vi "współrzedne geograficzne na UTM.vi"(0 "Położenie robota - długość geograficzna":dbl=44.0 format="%#_19g", 2 "Położenie robota - szerokość geograficzna":dbl=73.0 format="%#_19g", 3 "a":dbl=6378137.0 format="%_20g", 5 "b":dbl=6356752.3142452 format="%_20f") -> (6 "Strefa":string, 7 "E":dbl format="%.20g", 8 "N":dbl format="%.20g")   [LabVIEW 2015, in "Biblioteka moduł map v3.lvlib" / "Konwersja wsp.lvlib" / "UTM.lvlib"]
doc: "Jako argumenty przyjmowane są współrzędne w stopniach dziesiętnych. Domyslnie konwersja jest dokonywana dla współrzędnych w odwzorowaniu WGS84. Chcąc zastosować inne odwzorowanie Ziemi należy zmienić parametry geoidy (a,b).\nNa wyjscciu otrzymujemy strefę w pozycjonowaniu UTM oraz położenie N i E ( nie są to odpowiedniki kierunku północ, wschód). \n\nNie uwzględnoine zostały nierównomierne strefy: 31X, 33X, 35X, 37X, 31V, 32V dlatego dla tych obszarów nie powinno się stosować tego algorytmu. Dodatkowo nie wolno go stosować dla współrzędnych geograficznych znajdujących się poza zakresem 84 stopni N i 80 stopni S."
uses:
  UTM.lvlib
  Konwersja na UTM/Konwersja na UTM.lvlib
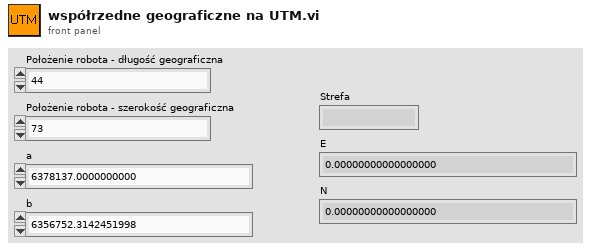
[diagram p1: front panel]
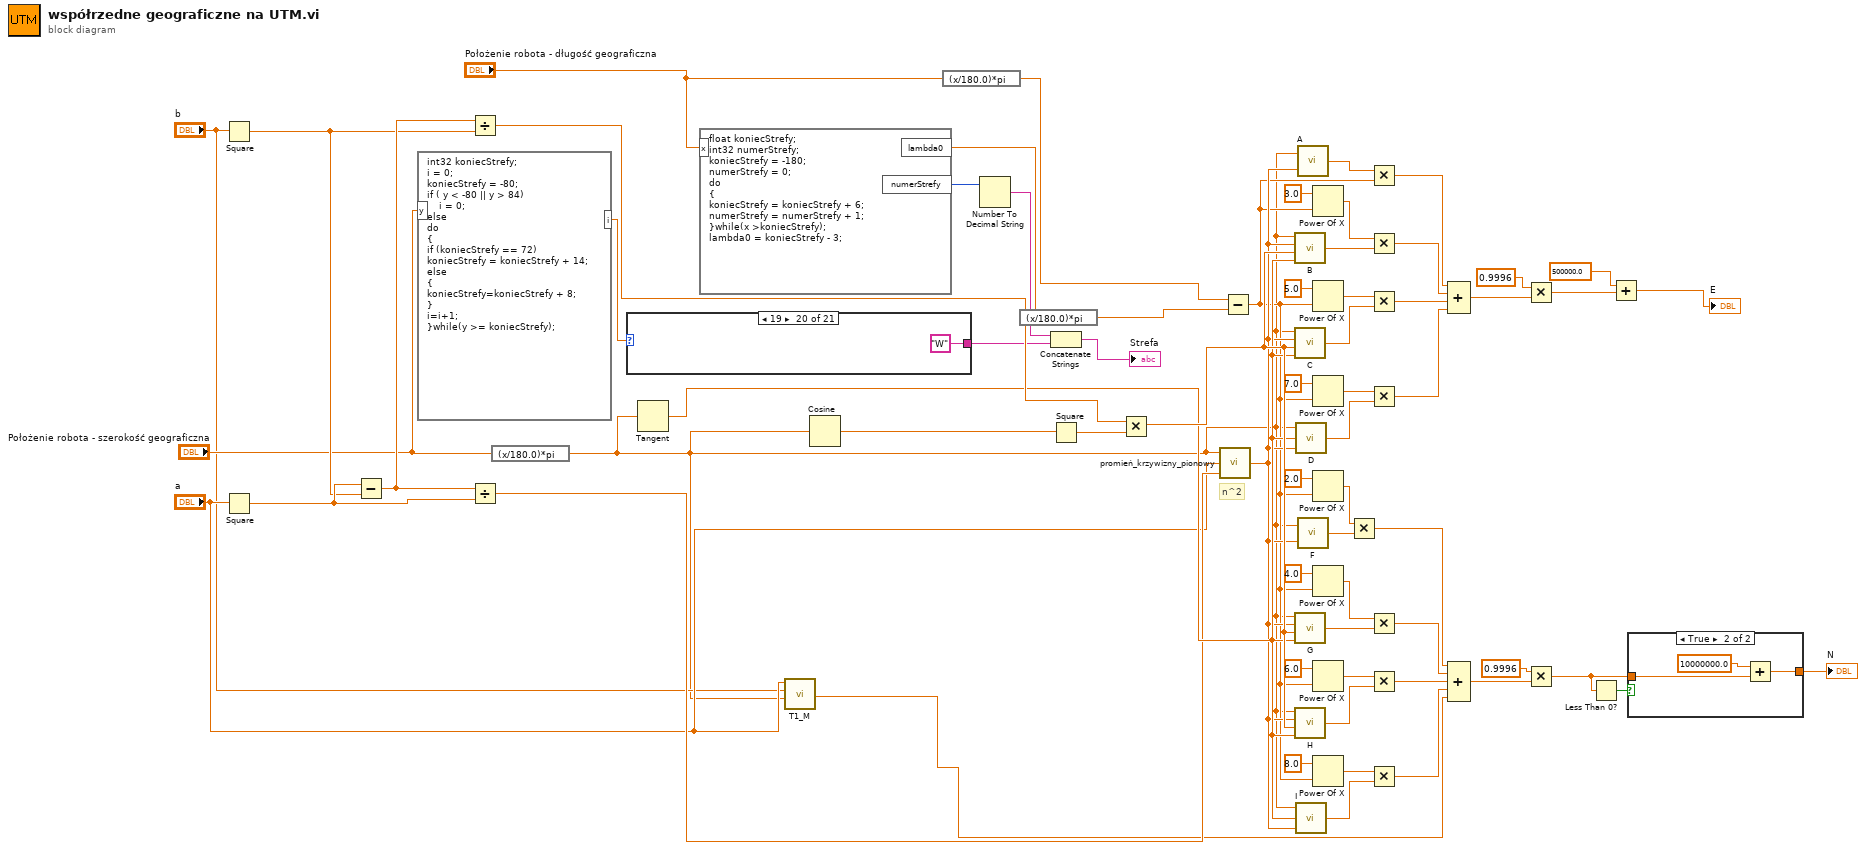
[diagram p0: block diagram]
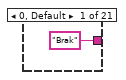
[diagram p3: hidden frame]
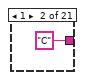
[diagram p4: hidden frame]
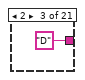
[diagram p5: hidden frame]
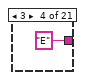
[diagram p6: hidden frame]
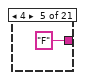
[diagram p7: hidden frame]
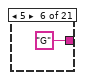
[diagram p8: hidden frame]
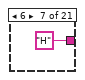
[diagram p9: hidden frame]
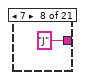
[diagram p10: hidden frame]
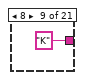
[diagram p11: hidden frame]
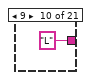
[diagram p12: hidden frame]
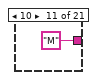
[diagram p13: hidden frame]
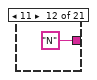
[diagram p14: hidden frame]
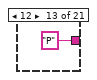
[diagram p15: hidden frame]
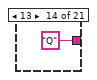
[diagram p16: hidden frame]
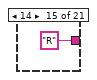
[diagram p17: hidden frame]
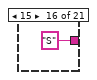
[diagram p18: hidden frame]
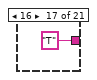
[diagram p19: hidden frame]
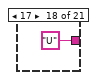
[diagram p20: hidden frame]
diagram:
  # "n^2"
  n1 = Square(x="b") -> (x^2=w63:dbl)
  n2 = Square(x="a") -> (x^2=w64:dbl)
  n3 = Subtract(x=w64, y=w63) -> (x-y=w65:dbl)
  n4 = formula code="int32 koniecStrefy;\ni = 0;\nkoniecStrefy = -80;\nif ( y < -80 || y > 84)\n    i = 0;\nelse\ndo\n{\nif (koniecStrefy == 72)\nkoniecStrefy = koniecStrefy + 14;\nelse\n{\nkoniecStrefy=koniecStrefy + 8;\n}\ni=i+1;\n}while(y >= koniecStrefy);"("y"="Położenie robota - szerokość geograficzna") -> ("i"=w16:dbl)
  n5 = Divide(x=w65, y=w63) -> (x/y=w60:dbl)
  n6 = Divide(x=w65, y=w64) -> (x/y=w54:dbl)
  n7 = expression code="(x/180.0)*pi" ("degrees to radians")("Położenie robota - szerokość geograficzna") -> (w2:dbl)
  n8 = case shown="19" w16 {
    tunnel: ["Brak" "C" "D" "E" "F" "G" "H" "J" "K" "L" "M" "N" "P" "Q" "R" "S" "T" "U" "V" "W" "X"] -> w14
    frame 0, Default {
    }
    frame 1 {
    }
    frame 2 {
    }
    frame 3 {
    }
    frame 4 {
    }
    frame 5 {
    }
    frame 6 {
    }
    frame 7 {
    }
    frame 8 {
    }
    frame 9 {
    }
    frame 10 {
    }
    frame 11 {
    }
    frame 12 {
    }
    frame 13 {
    }
    frame 14 {
    }
    frame 15 {
    }
    frame 16 {
    }
    frame 17 {
    }
    frame 18 {
    }
    frame 19 {
    }
    frame 20 {
    }
  }
  n9 = Tangent(1:w2) -> (0:w56:dbl)
  n10 = formula code="float koniecStrefy;\nint32 numerStrefy;\nkoniecStrefy = -180;\nnumerStrefy = 0;\ndo\n{\nkoniecStrefy = koniecStrefy + 6;\nnumerStrefy = numerStrefy + 1;\n}while(x >koniecStrefy);\nlambda0 = koniecStrefy - 3;"("x"="Położenie robota - długość geograficzna") -> ("lambda0"=w24:dbl, "numerStrefy"=w15:i32)
  n11 = call "T1_M.vi"("a"="a", "b"="b", "fi"=w2) -> ("T1_M"=w1:dbl)  [unwired: 5 in]
  n12 = Cosine(x=w2) -> (cos(x)=w58:dbl)
  n13 = expression code="(x/180.0)*pi" ("degrees to radians")("Położenie robota - długość geograficzna") -> (w61:dbl)
  n14 = Number To Decimal String(number=w15) -> (decimal integer string=w13:string)  [unwired: 1 in]
  n15 = expression code="(x/180.0)*pi" ("degrees to radians")(w24) -> (w62:dbl)
  n16 = Concatenate Strings(w13, w14) -> (→"Strefa":string)
  n17 = Square(x=w58) -> (x^2=w59:dbl)
  n18 = Multiply(x=w60, y=w59) -> (x*y=w57:dbl)
  n19 = call "promień_krzywizny_pionowy.vi"("e^2"=w54, "a"="a", "fi[rad]"=w2) -> ("Promien krzywizny równoleżnika"=w55:dbl)  [unwired: 2 in]
  n20 = Subtract(x=w61, y=w62) -> (x-y=w27:dbl)
  n21 = call "B.vi"("t"=w56, "n^2"=w57, "Promien krzywizny południka"=w55, "fi[rad]"=w2) -> ("B"=w51:dbl)  [unwired: 2 in]
  n22 = call "C.vi"("t"=w56, "n^2"=w57, "Promien krzywizny południka [v]"=w55, "fi[rad]"=w2) -> ("C"=w43:dbl)  [unwired: 2 in]
  n23 = call "G.vi"("t"=w56, "n^2"=w57, "Promien krzywizny południka [v]"=w55, "fi[rad]"=w2) -> ("G"=w30:dbl)  [unwired: 2 in]
  n24 = call "H.vi"("t"=w56, "n^2"=w57, "Promien krzywizny południka [v]"=w55, "fi[rad]"=w2) -> ("H"=w29:dbl)  [unwired: 2 in]
  n25 = call "D.vi"("Promien krzywizny południka [v]"=w55, "t"=w56, "fi[rad]"=w2) -> ("D"=w42:dbl)
  n26 = call "I.vi"("Promien krzywizny południka [v]"=w55, "t"=w56, "fi[rad]"=w2) -> ("D"=w28:dbl)
  n27 = call "A.vi"("Promien krzywizny południka [v]"=w55, ">fi[rad]>"=w2) -> ("A"=w53:dbl)
  n28 = call "F.vi"("Promien krzywizny południka [v]"=w55, "fi[rad]"=w2) -> ("D"=w31:dbl)
  n29 = Power Of X(1:w27, 2:3.0 ("y")) -> (0:w50:dbl)
  n30 = Power Of X(1:w27, 2:5.0 ("y")) -> (0:w46:dbl)
  n31 = Power Of X(1:w27, 2:7.0 ("y")) -> (0:w45:dbl)
  n32 = Power Of X(1:w27, 2:2.0 ("y")) -> (0:w33:dbl)
  n33 = Power Of X(1:w27, 2:4.0 ("y")) -> (0:w34:dbl)
  n34 = Power Of X(1:w27, 2:6.0 ("y")) -> (0:w37:dbl)
  n35 = Power Of X(1:w27, 2:8.0 ("y")) -> (0:w38:dbl)
  n36 = Multiply(x=w33, y=w31) -> (x*y=w23:dbl)
  n37 = Multiply(x=w53, y=w27) -> (x*y=w52:dbl)
  n38 = Multiply(x=w50, y=w51) -> (x*y=w48:dbl)
  n39 = Multiply(x=w46, y=w43) -> (x*y=w41:dbl)
  n40 = Multiply(x=w45, y=w42) -> (x*y=w40:dbl)
  n41 = Multiply(x=w34, y=w30) -> (x*y=w22:dbl)
  n42 = Multiply(x=w37, y=w29) -> (x*y=w21:dbl)
  n43 = Multiply(x=w38, y=w28) -> (x*y=w20:dbl)
  n44 = Compound Arithmetic op=ADD(w52, w48, w41, w40) -> (w10:dbl)
  n45 = Compound Arithmetic op=ADD(w23, w22, w21, w20, w1) -> (w25:dbl)
  n46 = Multiply(x=0.9996, y=w10) -> (x*y=w9:dbl)
  n47 = Multiply(x=0.9996, y=w25) -> (x*y=w18:dbl)
  n48 = Less Than 0?(x=w18) -> (x < 0?=w6:bool)
  n49 = Add(x=500000.0, y=w9) -> (x+y=→"E":dbl)
  n50 = case shown="True" w6 {
    tunnel: [w87 w89] -> w19
    tunnel: w18 -> [w87 w90]
    frame False {
    }
    frame True {
      n51 = Add(x=10000000.0, y=w90) -> (x+y=w89:dbl)
    }
  }
  "N" <- w19
